vi "Lifter_main.vi"() -> ()   [LabVIEW 2019]
uses:
  LifterSUBVis/Motor Class/Lifter_motor.lvclass
panel:
  out "Step Count":i32
  out "EOS BOS Data":bool
  out "Current insert in the fridge":string
  out "Insert used to calibration":string
  out "Calibration date":string
  out "Motor Speed (rev/s)":dbl
  out "LifterVelocity (mm/s)":dbl
  out "Status bar":string
  out "Moving status":bool
  out "Motor Running":bool
  out "Main Loop Running":bool
  in  "Move to cup abs":bool caption="Move"
  in  "Possition selector":T1(radio)
  in  "stop":bool
  out "chart_temp":waveform(dbl)[](graph)=[{"t0"=timestamp(3772890114.31303 s since 1904-01-01), "dt"=1.0, "Y"=[0.8687935985565186]}, {"t0"=timestamp(3772890114.31303 s since 1904-01-01), "dt"=1.0, "Y"=[86.87935985565186]}, {"t0"=timestamp(3772890114.31303 s since 1904-01-01), "dt"=1.0, "Y"=[30.48853325313992]}, {"t0"=timestamp(3772890114.31303 s since 1904-01-01), "dt"=1.0, "Y"=[303.6385332531399]}]
  out "Step Distance(mm)":dbl
  out "Pot Distance (mm)":dbl format="%#_5g"
  out "L. Limit":bool
  out "U.Limmit":bool
  out "Top":bool
  out "Middle":bool
  out "Bottom":bool
  out "Anneal":bool
  out "Home":bool
  out "Pot":dbl(slide) scale=280.0..-2.0
  out "Possition":dbl(slide) scale=280.0..-2.0
  in  "Show Advance Settings":bool
  in  "Advance Control":enum32{"Page 1", "Beam allignment setup "}(tab)
  in  "Manual Motor direction":bool
  in  "Move to save zone":bool
  in  "Reset Zero":bool
  in  "Up":bool
  in  "Down":bool
  in  "Fine Adjustments (0.005 mm)":dbl min=0.0 max=10.0 step=0.005 format="%#_4g"
  in  "Backlash correction":bool=TRUE
  out "Pot- Step":dbl
  out "ADC Voltage":dbl format="%.5f"
  in  "Move":bool
  in  "Set Velocity":bool
  in  "Set Velocity (mm/s)":dbl min=0.0 max=15.0
  in  "Record data":bool=TRUE
  in  "Remote port":u16=7776
  in  "IP Address":string="192.168.24.142"
  out "Switch Value":dbl
  in  "Data recording interval(ms)":u32=2000
  out "Data wright time (ms)":u32
  in  "Load insert parameters":bool
  in  "initialize the beam allignmet process":bool
  in  "Update newloca tion":bool
  in  "Update the lifter profile":bool
  in  "Insert name":enum16{"Insert #1", "Insert #2", "CALIB_INSERT"}(ring)
  in  "Select the cup":T2(radio)=enum."Bottom Cup on Beam"
  out "Beam alignment is running":bool
  out "New lifter configs_1":dbl[](array[numeric]) caption="Updated lifter configs"
  out "Insert Name_1":string
  out "New lifter configs_2":dbl[](array[numeric]) caption="Updated lifter configs"
  out "Insert Name_2":string
  out "Current insert-lifter config":dbl[](array[numeric]) caption="Updated lifter configs"
  out "Current insert":string
  out "error out":errorcluster
  in  "Exit VI":bool
  # "E-1039 Target Lifter System"
  # "Status"
  # "Possition Controlls"
  # "Cup Possition"
  # "Pot"
  # "Step"
  # "Communication Settings"
  # "Ignore POT and move"
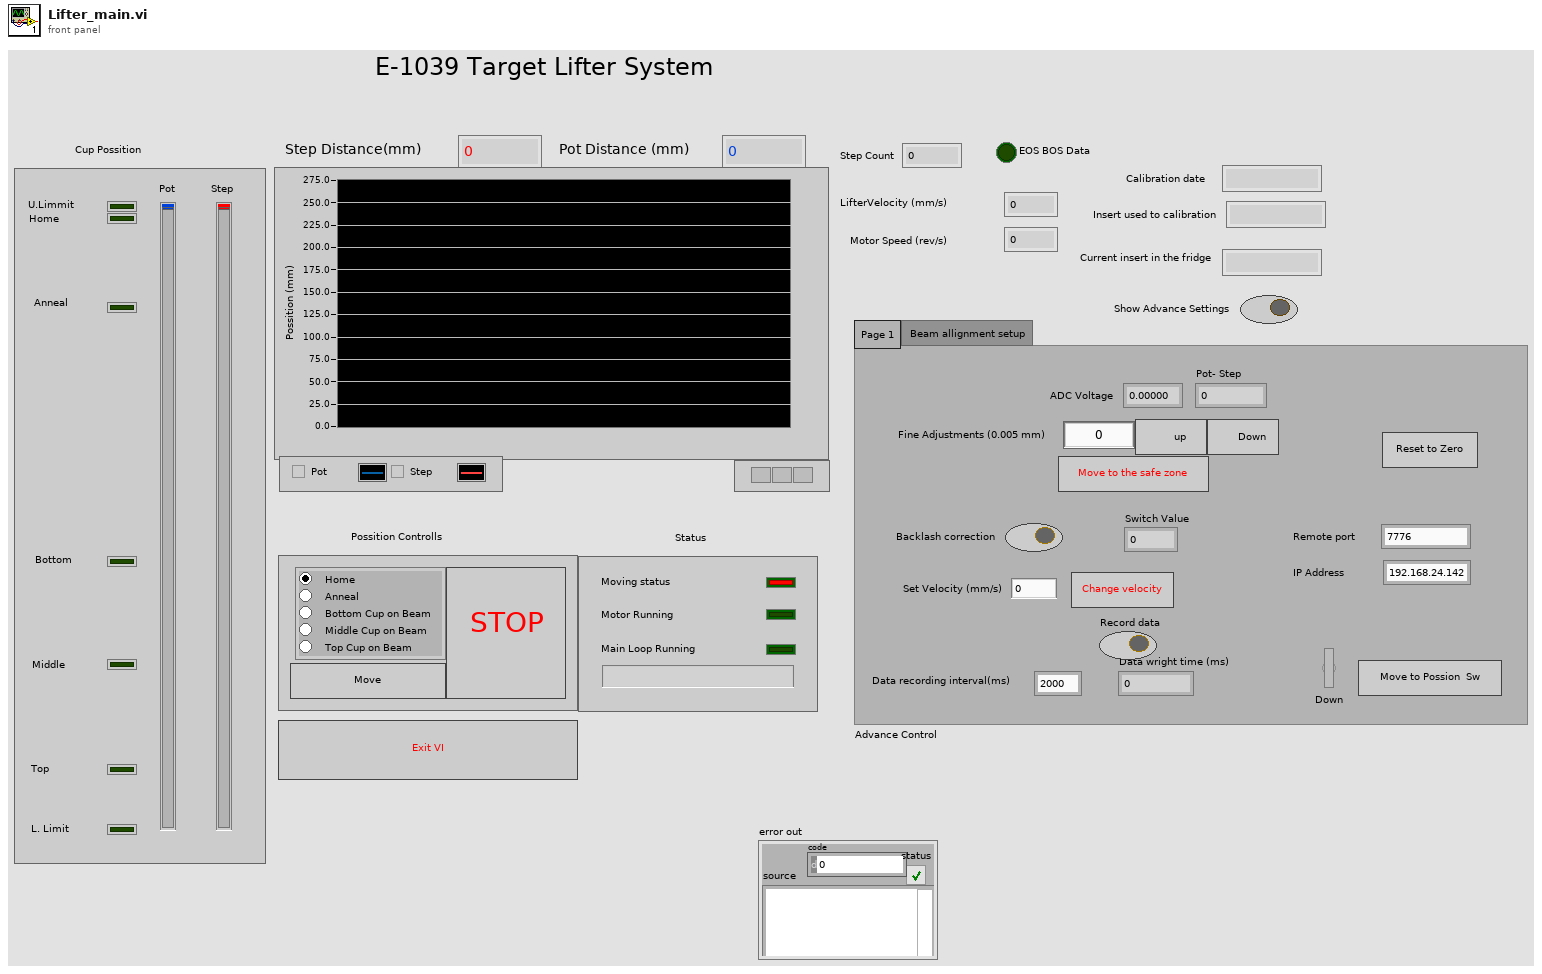
[diagram p1: front panel]
types:
  T1 = enum32{"Home", "Anneal", "Bottom Cup on Beam", "Middle Cup on Beam", "Top Cup on Beam"}
  T2 = enum32{"No Selection", "Bottom Cup on Beam", "Middle Cup on Beam", "Top Cup on Beam"}
  T3 = enum8{"Enabled", "Disabled", "Disabled and Grayed Out"}
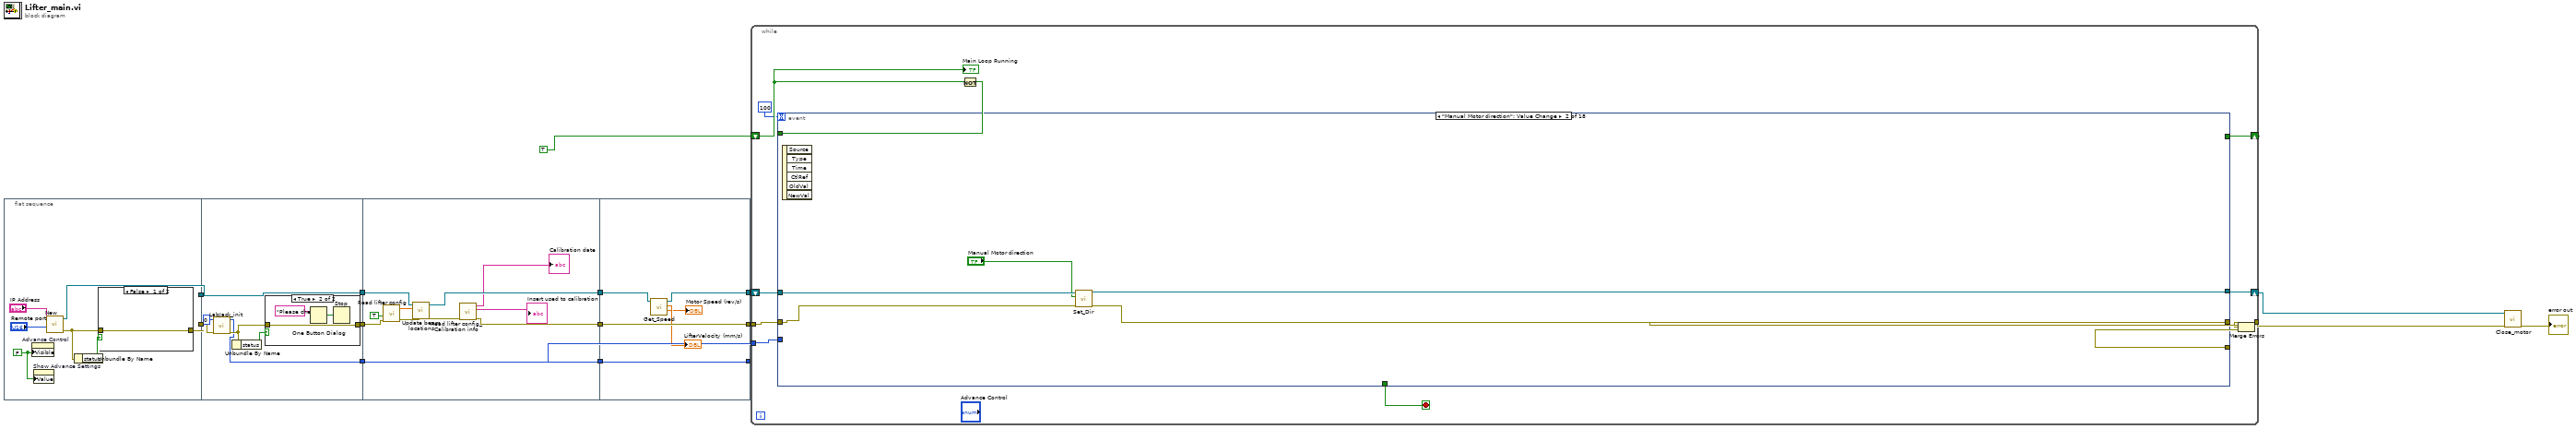
[diagram p0: block diagram]
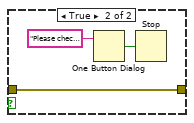
[diagram p2: hidden frame]
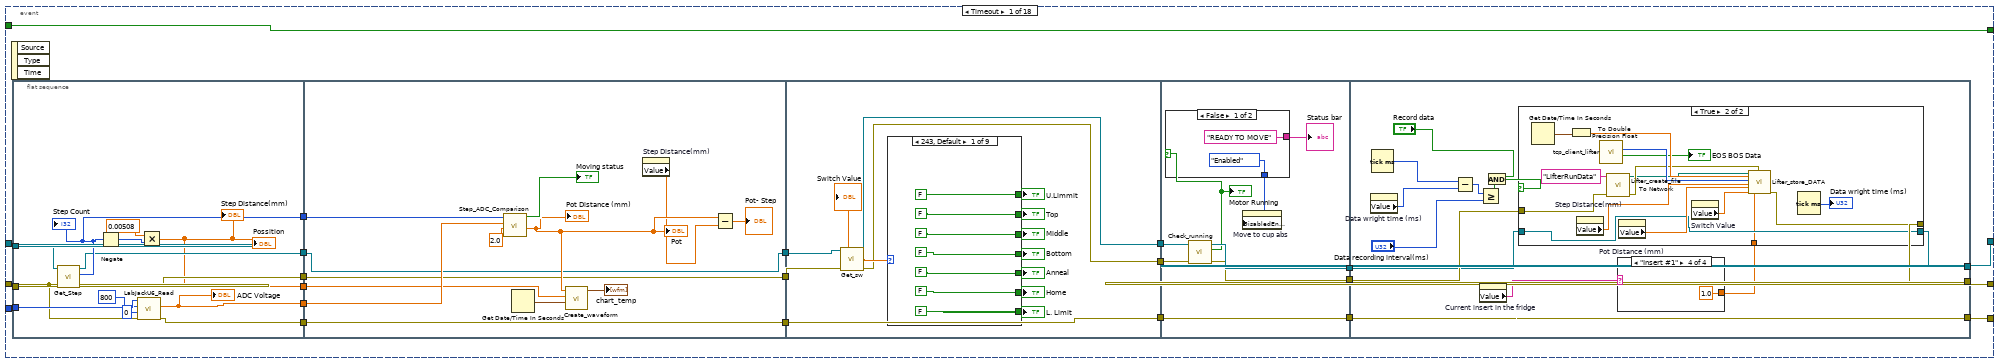
[diagram p4: hidden frame]
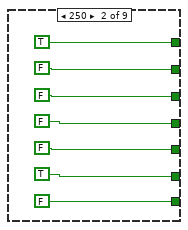
[diagram p5: hidden frame]
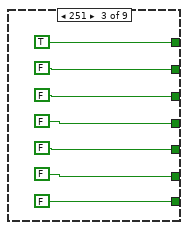
[diagram p6: hidden frame]
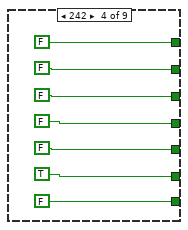
[diagram p7: hidden frame]
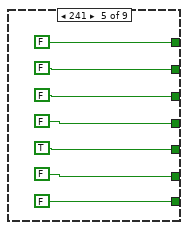
[diagram p8: hidden frame]
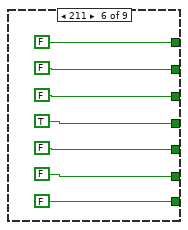
[diagram p9: hidden frame]
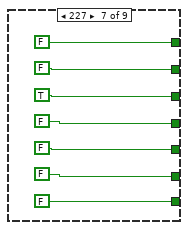
[diagram p10: hidden frame]
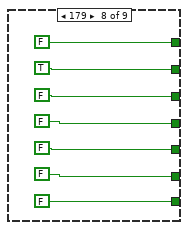
[diagram p11: hidden frame]
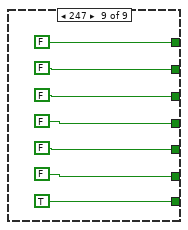
[diagram p12: hidden frame]
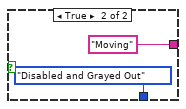
[diagram p13: hidden frame]
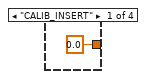
[diagram p14: hidden frame]
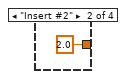
[diagram p15: hidden frame]
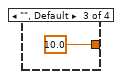
[diagram p16: hidden frame]
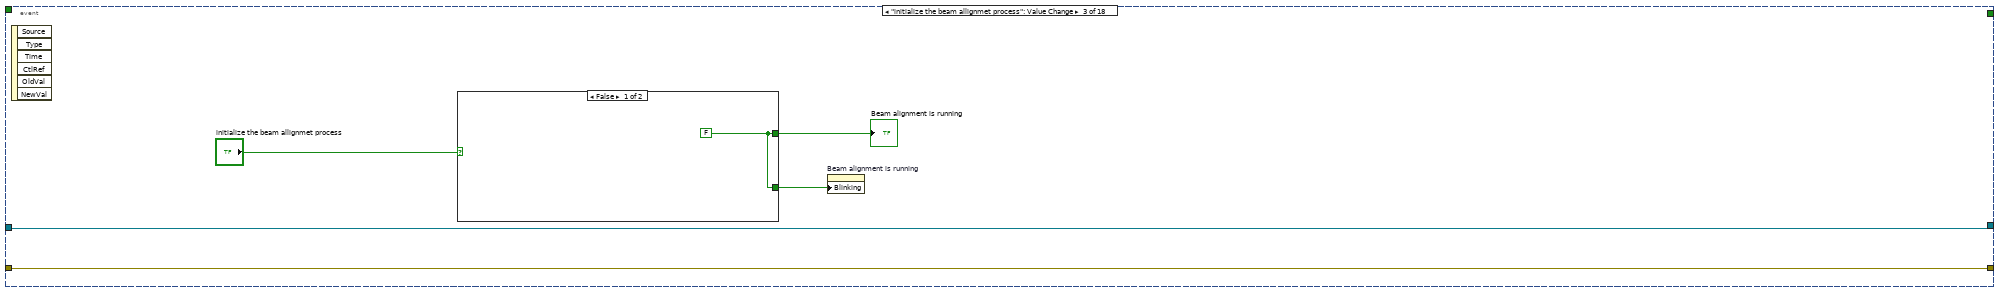
[diagram p18: hidden frame]
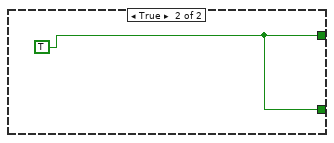
[diagram p19: hidden frame]
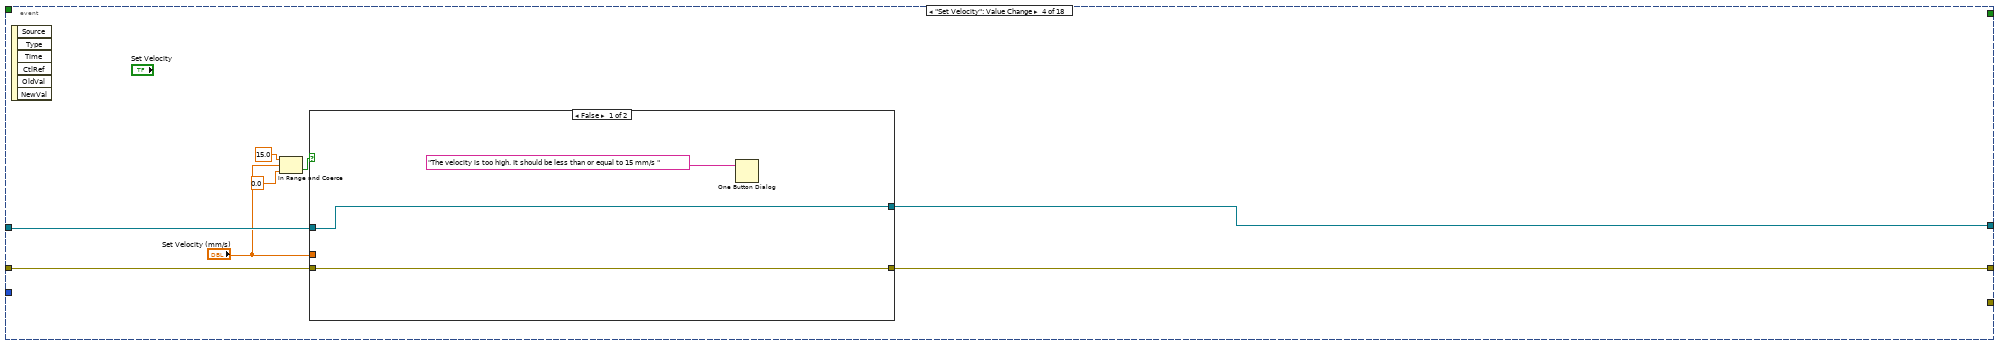
[diagram p20: hidden frame]
diagram:
  n1 = flat-sequence {
    tunnel: [w21] -> w13
    tunnel: [w17] -> w10
    tunnel: w13 -> [w30]
    tunnel: w10 -> [w27]
    tunnel: [w31] -> w6
    tunnel: [w28] -> w4
    tunnel: [w27] -> w2
    tunnel: w6 -> [w47]
    tunnel: [w40] -> w5
    tunnel: w4 -> [w48]
    tunnel: [w48] -> w3
    tunnel: w2 -> [w45]
    tunnel: [w44] -> w1
    tunnel: [w51] -> w11
    tunnel: [w53] -> w12
    tunnel: [w54] -> w14
    tunnel: w5 -> [w54]
    tunnel: w3 -> [w53]
    tunnel: w1 -> [w52]
    frame #0 {
      w16 = FALSE ("Visible")
      n2 = property on="Advance Control" class="TabCtl (strict)"("Visible"=w16) -> ()  [unwired: 2 in, 2 out]
      n3 = property on="Show Advance Settings" class="Bool (strict)"("Value"=w16) -> ()  [unwired: 2 in, 2 out]
      n4 = call "New.vi"("remote port or service name"="Remote port", "address"="IP Address") -> ("error out"=w18:errorcluster, "Lifter_motor out"=w17:refnum<class "Lifter_motor.lvclass">)  [unwired: 8 in]
      n5 = Unbundle By Name(w18) -> ("status"=w22:bool)
      n6 = case shown="False" w22 {
        tunnel: [w23 w25] -> w21
        tunnel: w18 -> [w23 w25]
        frame False {
        }
        frame True {
          n7 = One Button Dialog(message="Please check the motor driver. VI is closing ") -> (true=w24:bool)  [unwired: 1 in]
          n8 = Stop(stop? (T)=w24) -> ()
        }
      }
    }
    frame #1 {
      n9 = call "LabJack_init.vi"("error in"=w30, "Positive Channel #"=0) -> ("error out"=w33:errorcluster, "Handle Out"=w28:i32)  [unwired: 7 in, 1 out]
      n10 = Unbundle By Name(w33) -> ("status"=w32:bool)
      n11 = case shown="True" w32 {
        tunnel: [w34 w36] -> w31
        tunnel: w33 -> [w34 w36]
        frame False {
        }
        frame True {
          n12 = One Button Dialog(message="Please check the ADC. VI is closing ") -> (true=w35:bool)  [unwired: 1 in]
          n13 = Stop(stop? (T)=w35) -> ()
        }
      }
    }
    frame #2 {
      n14 = call "Read lifter config.vi"("Default"=TRUE, "error in (no error)"=w47) -> ("Lifter locations array"=w43:dbl[], "error out"=w46:errorcluster)  [unwired: 5 in]
      n15 = call "Update beam locations.vi"("error in (no error)"=w46, "New cup location"=w43, "Lifter_motor in"=w45) -> ("error out"=w41:errorcluster, "Lifter_motor out"=w44:refnum<class "Lifter_motor.lvclass">)  [unwired: 7 in]
      n16 = call "Read lifter config_Calibration info.vi"("error in (no error)"=w41) -> ("error out"=w40:errorcluster, "Insert"=→"Insert used to calibration":string, "Date"=→"Calibration date":string)  [unwired: 4 in]
    }
    frame #3 {
      n17 = call "Get_Speed.vi"("Lifter_motor in"=w52) -> ("Motor Speed (rev/s)"=→"Motor Speed (rev/s)":dbl, "Target Velocity (mm/s)"=→"LifterVelocity (mm/s)":dbl, "Lifter_motor out"=w51:refnum<class "Lifter_motor.lvclass">)  [unwired: 7 in, 1 out]
    }
  }
  n18 = while {
    tunnel: w14 -> [w65]
    shift-right: [w64] -> _
    shift-left: TRUE ("Main Loop Running") -> [w63]
    tunnel: w12 -> [w60]
    tunnel: [w56] -> w9
    shift-right: [w55] -> w7
    shift-left: w11 -> [w59]
    stop <- w66 stop-if-true
    n19 = Not(x=w63) -> (.not. x?=w62:bool)
    n20 = event shown="[1] \"Manual Motor direction\": Value Change" {
      selector: _ -> [_ _ _ _ _ _ _ _ _ _ _ _ _ _ _ _ _ _]
      dyn-events: _ -> [_ _ _ _ _ _ _ _ _ _ _ _ _ _ _ _ _ _]
      timeout: 100 -> [_ _ _ _ _ _ _ _ _ _ _ _ _ _ _ _ _ _]
      tunnel: [_ _ _ _ _ _ _ _ _ _ _ _ _ _ _ _ w391 _] -> w66
      tunnel: w65 -> [w88 w241 w244 w256 w277 w278 w288 w290 w300 w322 w362 w363 w371 w378 w383 w389 w390 w406]
      tunnel: w62 -> [w87 _ _ _ _ _ _ _ _ _ _ _ _ _ _ _ _ _]
      tunnel: [w87 _ _ _ _ _ _ _ _ _ _ _ _ _ _ _ _ _] -> w64
      tunnel: w60 -> [w78 _ _ _ _ _ _ _ _ _ _ _ _ _ _ _ _ _]
      tunnel: [w81 w239 w244 w254 w271 w278 w282 w289 w299 w322 w361 w364 w370 w377 w382 w388 w390 w407] -> w57
      tunnel: w59 -> [w82 w242 w245 w257 w272 w279 w284 w293 w302 w323 w359 w367 w372 w375 w380 w387 w393 w405]
      tunnel: [w69 w240 w245 w255 w270 w279 w283 w292 w298 w323 w360 w365 w369 w376 w381 w386 w393 w404] -> w55
      tunnel: [w74 _ _ _ _ _ _ _ _ _ w348 _ _ _ _ _ _ _] -> w58
      event Timeout {
        n21 = event-data() -> ()  [unwired: 1 in, 3 out]
        n22 = flat-sequence {
          tunnel: w88 -> [w96]
          tunnel: [w101] -> w86
          tunnel: [w100] -> w83
          tunnel: w82 -> [w99]
          tunnel: [w97] -> w80
          tunnel: [w91] -> w79
          tunnel: w78 -> [w98]
          tunnel: [w95] -> w75
          tunnel: [w90] -> w70
          tunnel: w86 -> [w107]
          tunnel: w83 -> [w102]
          tunnel: w80 -> [w103]
          tunnel: w79 -> [w112]
          tunnel: [w111] -> w76
          tunnel: w75 -> [w111]
          tunnel: w70 -> [w108]
          tunnel: [w103] -> w68
          tunnel: [w102] -> w67
          tunnel: [w118] -> w85
          tunnel: [w117] -> w84
          tunnel: [w115] -> w77
          tunnel: w76 -> [w115]
          tunnel: w68 -> [w120]
          tunnel: w67 -> [w116]
          tunnel: w85 -> [w198]
          tunnel: w84 -> [w197]
          tunnel: w77 -> [w194]
          tunnel: [w196] -> w73
          tunnel: [w195] -> w72
          tunnel: [w194] -> w71
          tunnel: [w216] -> w74
          tunnel: [w215] -> w81
          tunnel: [w205] -> w69
          tunnel: w73 -> [w206]
          tunnel: w72 -> [w214]
          tunnel: w71 -> [w216]
          frame #0 {
            n23 = call "Get_Step.vi"("error in (no error)"=w96, "Lifter_motor in"=w99) -> ("error out"=w97:errorcluster, "Step Count"=w101:i32, "Lifter_motor out"=w100:refnum<class "Lifter_motor.lvclass">)  [unwired: 7 in]
            "Step Count" <- w101
            n24 = Negate(x=w101) -> (-x=w93:i32)
            n25 = call "LabJackU6_Read.vi"("error in"=w96, "Positive Channel #"=0, "n_samples"=800, "Handle In"=w98) -> ("error out"=w95:errorcluster, "Mean ADC Voltage"=w91:dbl)  [unwired: 4 in, 2 out]
            "ADC Voltage" <- w91
            n26 = Multiply(x=0.00508, y=w93) -> (x*y=w90:dbl)
            "Possition" <- w90
            "Step Distance(mm)" <- w90
          }
          frame #1 {
            n27 = call "Step_ADC_Comparison.vi"("Range(mm)"=2.0, "ADC Voltage"=w112, "Steps"=w107) -> ("ADC Distance (mm)"=w106:dbl, "In range"=→"Moving status":bool)  [unwired: 5 in, 1 out]
            "Pot Distance (mm)" <- w106
            "Pot" <- w106
            n28 = Get Date/Time In Seconds() -> (seconds since 1Jan1904=w109:timestamp)
            n29 = call "Create_waveform.vi"("time"=w109, "Step Pos"=w108, "ADC Pos"=w106) -> ("waveform_array"=→"chart_temp":waveform(dbl)[])  [unwired: 8 in]
            n30 = property on="Step Distance(mm)" class="DigNum (strict)"() -> ("Value"=w105:dbl)  [unwired: 2 in, 2 out]
            n31 = Subtract(x=w106, y=w105) -> (x-y=→"Pot- Step":dbl)
          }
          frame #2 {
            n32 = call-dynamic "Get_sw.vi"("error in (no error)"=w120, "Lifter_motor in"=w116) -> ("error out"=w118:errorcluster, "Switch Hex"=w119:dbl, "Lifter_motor out"=w117:refnum<class "Lifter_motor.lvclass">)  [unwired: 7 in]
            "Switch Value" <- w119
            n33 = case shown="243, Default" w119 {
              tunnel: [FALSE ("Lower Limit") TRUE ("Lower Limit") TRUE ("Lower Limit") FALSE ("Lower Limit") FALSE ("Lower Limit") FALSE ("Lower Limit") FALSE ("Lower Limit") FALSE ("Lower Limit") FALSE ("Lower Limit")] -> w127
              tunnel: [FALSE ("Lower Limit") FALSE ("Lower Limit") FALSE ("Lower Limit") FALSE ("Lower Limit") FALSE ("Lower Limit") FALSE ("Lower Limit") FALSE ("Lower Limit") TRUE ("Lower Limit") FALSE ("Lower Limit")] -> w126
              tunnel: [FALSE ("Lower Limit") FALSE ("Lower Limit") FALSE ("Lower Limit") FALSE ("Lower Limit") FALSE ("Lower Limit") FALSE ("Lower Limit") TRUE ("Lower Limit") FALSE ("Lower Limit") FALSE ("Lower Limit")] -> w125
              tunnel: [FALSE ("Lower Limit") FALSE ("Lower Limit") FALSE ("Lower Limit") FALSE ("Lower Limit") FALSE ("Lower Limit") TRUE ("Lower Limit") FALSE ("Lower Limit") FALSE ("Lower Limit") FALSE ("Lower Limit")] -> w124
              tunnel: [FALSE ("Lower Limit") FALSE ("Lower Limit") FALSE ("Lower Limit") FALSE ("Lower Limit") TRUE ("Lower Limit") FALSE ("Lower Limit") FALSE ("Lower Limit") FALSE ("Lower Limit") FALSE ("Lower Limit")] -> w123
              tunnel: [FALSE ("Lower Limit") TRUE ("Lower Limit") FALSE ("Lower Limit") TRUE ("Lower Limit") FALSE ("Lower Limit") FALSE ("Lower Limit") FALSE ("Lower Limit") FALSE ("Lower Limit") FALSE ("Lower Limit")] -> w122
              tunnel: [FALSE ("Lower Limit") FALSE ("Lower Limit") FALSE ("Lower Limit") FALSE ("Lower Limit") FALSE ("Lower Limit") FALSE ("Lower Limit") FALSE ("Lower Limit") FALSE ("Lower Limit") TRUE ("Lower Limit")] -> w121
              frame 243, Default {
              }
              frame 250 {
              }
              frame 251 {
              }
              frame 242 {
              }
              frame 241 {
              }
              frame 211 {
              }
              frame 227 {
              }
              frame 179 {
              }
              frame 247 {
              }
            }
            "L. Limit" <- w121
            "Home" <- w122
            "Bottom" <- w124
            "Middle" <- w125
            "Anneal" <- w123
            "Top" <- w126
            "U.Limmit" <- w127
          }
          frame #3 {
            n34 = call "Check_running.vi"("error in (no error)"=w198, "Lifter_motor in"=w197) -> ("error out"=w195:errorcluster, "Status"=w193:bool, "Lifter_motor out"=w196:refnum<class "Lifter_motor.lvclass">)  [unwired: 6 in, 1 out]
            "Motor Running" <- w193
            n35 = case shown="False" w193 {
              tunnel: [T3."Enabled" ("Disabled") T3."Disabled and Grayed Out" ("Disabled")] -> w192
              tunnel: ["READY TO MOVE" ("Status bar") "Moving" ("Status bar")] -> w191
              frame False {
              }
              frame True {
              }
            }
            "Status bar" <- w191
            n36 = property on="Move to cup abs" class="Bool (strict)"("DisabledEnum"=w192) -> ()  [unwired: 2 in, 2 out]
          }
          frame #4 {
            n37 = property on="Data wright time (ms)" class="DigNum (strict)"() -> ("Value"=w211:u32)  [unwired: 2 in, 2 out]
            n38 = Tick Count (ms)() -> (millisecond timer value=w213:u32)
            n39 = Subtract(x=w213, y=w211) -> (x-y=w212:u32)
            n40 = Greater Or Equal?(x=w212, y="Data recording interval(ms)") -> (x >= y?=w210:bool)
            n41 = property on="Current insert in the fridge" class="Str"() -> ("Value"=w204:string)  [unwired: 2 in, 2 out]
            n42 = And(x="Record data", y=w210) -> (x .and. y?=w209:bool)
            n43 = case shown="\"Insert #1\"" w204 {
              tunnel: [0.0 ("Insert Number") 2.0 ("Insert Number") 10.0 ("Insert Number") 1.0 ("Insert Number")] -> w203
              frame "CALIB_INSERT" {
              }
              frame "Insert #2" {
              }
              frame "", Default {
              }
              frame "Insert #1" {
              }
            }
            n44 = case shown="True" w209 {
              tunnel: w214 -> [w222 w225]
              tunnel: [w222 w233] -> w215
              tunnel: w206 -> [w221 w228]
              tunnel: [w221 w228] -> w205
              tunnel: w203 -> [_ w223]
              frame False {
              }
              frame True {
                n45 = Get Date/Time In Seconds() -> (seconds since 1Jan1904=w237:timestamp)
                n46 = To Double Precision Float(number=w237) -> (double precision float=w236:dbl)
                n47 = property on="Step Distance(mm)" class="DigNum (strict)"() -> ("Value"=w230:dbl)  [unwired: 2 in, 2 out]
                n48 = call "tcp_client_lifter.vi"() -> ("status"=→"EOS BOS Data":bool, "Spill ID"=w235:i32)  [unwired: 8 in, 2 out]
                n49 = call "Lifter_create_file To Network.vi"("error in (no error)"=w225, "File Name"="LifterRunData") -> ("error out"=w227:errorcluster, "dup path"=w226:path)  [unwired: 8 in]
                n50 = property on="Pot Distance (mm)" class="DigNum (strict)"() -> ("Value"=w229:dbl)  [unwired: 2 in, 2 out]
                n51 = property on="Switch Value" class="DigNum (strict)"() -> ("Value"=w234:dbl)  [unwired: 2 in, 2 out]
                n52 = call "Lifter_store_DATA.vi"("file path (dialog if empty)"=w226, "Time stamp"=w236, "Spill ID"=w235, "Step Distance"=w230, "Pot Disance"=w229, "Possition indicator switch"=w234, "Insert Number"=w223, "error in (no error)"=w227) -> ("error out"=w233:errorcluster)  [unwired: 10 in, 1 out]
                n53 = Tick Count (ms)() -> (millisecond timer value=→"Data wright time (ms)":u32)
              }
            }
          }
        }
      }
      event "Manual Motor direction": Value Change {
        n54 = event-data() -> ()  [unwired: 1 in, 6 out]
        n55 = call "Set_Dir.vi"("error in (no error)"=w241, "Direction"="Manual Motor direction", "Lifter_motor in"=w242) -> ("error out"=w239:errorcluster, "Lifter_motor out"=w240:refnum<class "Lifter_motor.lvclass">)  [unwired: 6 in, 1 out]
      }
      event "initialize the beam allignmet process": Value Change {
        n56 = event-data() -> ()  [unwired: 1 in, 6 out]
        n57 = case shown="False" "initialize the beam allignmet process" {
          tunnel: [w248 w249] -> w243
          tunnel: [w248 w249] -> w246
          frame False {
            w248 = FALSE ("Beam alignment is running")
          }
          frame True {
            w249 = TRUE ("Beam alignment is running")
          }
        }
        "Beam alignment is running" <- w243
        n58 = property on="Beam alignment is running" class="Bool (strict)"("Blinking"=w246) -> ()  [unwired: 2 in, 2 out]
      }
      event "Set Velocity": Value Change {
        n59 = event-data() -> ()  [unwired: 1 in, 6 out]
        n60 = In Range and Coerce(upper limit=15.0 ("lower limit"), x="Set Velocity (mm/s)", lower limit=0.0 ("upper limit")) -> (In Range?=w252:bool)  [unwired: 1 out]
        n61 = case shown="False" w252 {
          tunnel: w257 -> [w259 w269]
          tunnel: w256 -> [w260 w268]
          tunnel: [w259 w263] -> w255
          tunnel: [w260 w262] -> w254
          tunnel: "Set Velocity (mm/s)" -> [_ w261]
          frame False {
            n62 = One Button Dialog(message="The velocity is too high. It should be less than or equal to 15 mm/s ") -> ()  [unwired: 1 in, 1 out]
          }
          frame True {
            n63 = call "Set_velocity.vi"("error in (no error)"=w268, "Set Velocity (mm/s)"=w261, "Lifter_motor in"=w269) -> ("error out"=w267:errorcluster, "Lifter_motor out"=w266:refnum<class "Lifter_motor.lvclass">)  [unwired: 7 in]
            n64 = call "Get_Speed.vi"("error in (no error)"=w267, "Lifter_motor in"=w266) -> ("error out"=w262:errorcluster, "Motor Speed (rev/s)"=w264:dbl, "Target Velocity (mm/s)"=w265:dbl, "Lifter_motor out"=w263:refnum<class "Lifter_motor.lvclass">)  [unwired: 6 in]
            n65 = property on="Motor Speed (rev/s)" class="DigNum (strict)"("Value"=w264) -> ()  [unwired: 2 in, 2 out]
            n66 = property on="LifterVelocity (mm/s)" class="DigNum (strict)"("Value"=w265) -> ()  [unwired: 2 in, 2 out]
          }
        }
      }
      event "Move to save zone": Value Change {
        n67 = event-data() -> ()  [unwired: 1 in, 6 out]
        n68 = call "Step mm con.vi"("error in (no error)"=w277, "mm in"=91.054) -> ("error out"=w275:errorcluster, "step out"=w274:i32)  [unwired: 7 in, 1 out]
        n69 = Negate(x=w274) -> (-x=w273:i32)
        n70 = call "Move to Abs Step location.vi"("error in (no error)"=w275, "Absolute step location to move"=w273, "Lifter_motor in"=w272) -> ("error out"=w271:errorcluster, "Lifter_motor out"=w270:refnum<class "Lifter_motor.lvclass">)  [unwired: 6 in, 1 out]
      }
      event "Show Advance Settings": Value Change {
        n71 = event-data() -> ()  [unwired: 1 in, 6 out]
        n72 = property on="Advance Control" class="TabCtl (strict)"("Visible"="Show Advance Settings") -> ()  [unwired: 2 in, 2 out]
      }
      event "Move": Value Change {
        n73 = event-data() -> ()  [unwired: 1 in, 6 out]
        n74 = property on="Step Count" class="DigNum (strict)" props=["Value"]() -> ()  [unwired: 2 in, 3 out]
        n75 = property on="Pot Distance (mm)" class="DigNum (strict)"() -> ("Value"=w286:dbl)  [unwired: 2 in, 2 out]
        n76 = property on="Step Distance(mm)" class="DigNum (strict)"() -> ("Value"=w281:dbl)  [unwired: 2 in, 2 out]
        n77 = property on="Moving status" class="Bool (strict)"() -> ("Value"=w285:bool)  [unwired: 2 in, 2 out]
        n78 = call "Move To Pos.vi"("Lifter_motor in"=w284, "Step In range"=w285, "Step Distance"=w281, "ADC distance"=w286, "Possition selector"="Possition selector", "error in (no error)"=w288) -> ("Lifter_motor out"=w283:refnum<class "Lifter_motor.lvclass">, "error out"=w282:errorcluster)  [unwired: 7 in, 1 out]
      }
      event "Select the cup": Value Change {
        n79 = event-data() -> ()  [unwired: 1 in, 6 out]
        n80 = call "View  beam possitions.vi"("error in (no error)"=w290, "Beam on cup"="Select the cup", "Lifter_motor in"=w293) -> ("error out"=w289:errorcluster, "Lifter_motor out"=w292:refnum<class "Lifter_motor.lvclass">)  [unwired: 6 in, 1 out]
      }
      event "Update the lifter profile": Value Change {
        n81 = event-data() -> ()  [unwired: 1 in, 6 out]
        n82 = property on="Update newloca tion" class="Bool"("DisabledEnum"=T3."Enabled" ("Disabled")) -> ()  [unwired: 2 in, 2 out]
        n83 = property on="Step Distance(mm)" class="DigNum (strict)"() -> ("Value"=w308:dbl)  [unwired: 2 in, 2 out]
        n84 = property on="Select the cup" class="RadioBtnsControl (strict)"() -> ("Value"=w309:T2)  [unwired: 2 in, 2 out]
        n85 = call "Generate_insert cup locations .vi"("Lifter reading (mm)"=w308, "Select the cup"=w309) -> ("Top"=w305:dbl, "Middle"=w306:dbl, "Bottom"=w307:dbl)  [unwired: 7 in]
        n86 = call "Write to lifter config.vi"("Insert name"="Insert name", "Bottom"=w307, "Middle"=w306, "Top"=w305, "error in (no error)"=w300) -> ("error out"=w303:errorcluster)  [unwired: 9 in, 1 out]
        n87 = call "Write to lifter config.vi"("Default"=TRUE, "Bottom"=w307, "Middle"=w306, "Top"=w305, "error in (no error)"=w303) -> ("Cup locations"=w294:dbl[], "error out"=w301:errorcluster)  [unwired: 9 in]
        "Current insert-lifter config" <- w294
        n88 = property on="Insert name" class="Enum (strict)"() -> ("Strings []"=w296:string[])  [unwired: 2 in, 2 out]
        n89 = Index Array(array=w296, index="Insert name") -> (element=→"Current insert":string)
        n90 = call "Update beam locations.vi"("error in (no error)"=w301, "New cup location"=w294, "Lifter_motor in"=w302) -> ("error out"=w299:errorcluster, "Lifter_motor out"=w298:refnum<class "Lifter_motor.lvclass">)  [unwired: 7 in]
      }
      event "Update newloca tion": Value Change {
        n91 = event-data() -> ()  [unwired: 1 in, 6 out]
        n92 = property on="Insert name" class="Enum (strict)"() -> ("Value"=w317:enum16{"Insert #1", "Insert #2", "CALIB_INSERT"})  [unwired: 2 in, 2 out]
        n93 = call "Read inserts profiles.vi"("Insert name"=w317) -> ("error out"=w344:errorcluster, "top cup length"=w330:dbl)  [unwired: 7 in]
        n94 = Increment(x=w317) -> (x+1=w315:enum16{"Insert #1", "Insert #2", "CALIB_INSERT"})
        n95 = call "Read inserts profiles.vi"("error in (no error)"=w344, "Insert name"=w315) -> ("error out"=w342:errorcluster, "top cup length"=w343:dbl)  [unwired: 6 in]
        n96 = Subtract(x=w330, y=w343) -> (x-y=w340:dbl)
        n97 = property on="Insert name" class="Enum (strict)"() -> ("Strings []"=w316:string[])  [unwired: 2 in, 2 out]
        n98 = call "Read lifter config.vi"("Insert name"=w317, "error in (no error)"=w342) -> ("Lifter locations array"=w341:dbl[], "error out"=w332:errorcluster)  [unwired: 5 in]
        n99 = Add(x=w340, y=w341) -> (x+y=w339:dbl[])
        "New lifter configs_1" <- w339
        n100 = Index Array(array=w316, index=w315) -> (element=→"Insert Name_1":string)
        n101 = Index Array(array=w339, index #1=0 ("index")) -> (element #1=w338:dbl, element #2=w337:dbl, element #3=w336:dbl)  [unwired: 2 in]
        n102 = call "Write to lifter config.vi"("Insert name"=w315, "Bottom"=w338, "Middle"=w337, "Top"=w336) -> ()  [unwired: 10 in, 2 out]
        n103 = Increment(x=w315) -> (x+1=w312:enum16{"Insert #1", "Insert #2", "CALIB_INSERT"})
        n104 = call "Read inserts profiles.vi"("error in (no error)"=w332, "Insert name"=w312) -> ("error out"=w331:errorcluster, "top cup length"=w335:dbl)  [unwired: 6 in]
        n105 = Subtract(x=w330, y=w335) -> (x-y=w333:dbl)
        n106 = property on="Insert name" class="Enum (strict)"() -> ("Strings []"=w313:string[])  [unwired: 2 in, 2 out]
        n107 = call "Read lifter config.vi"("Insert name"=w317, "error in (no error)"=w331) -> ("Lifter locations array"=w334:dbl[], "error out"=w320:errorcluster)  [unwired: 5 in]
        n108 = Index Array(array=w313, index=w312) -> (element=→"Insert Name_2":string)
        n109 = Add(x=w333, y=w334) -> (x+y=w326:dbl[])
        "New lifter configs_2" <- w326
        n110 = Index Array(array=w326, index #1=0 ("index")) -> (element #1=w327:dbl, element #2=w328:dbl, element #3=w329:dbl)  [unwired: 2 in]
        n111 = call "Write to lifter config.vi"("Insert name"=w312, "Bottom"=w327, "Middle"=w328, "Top"=w329, "error in (no error)"=w320) -> ("error out"=w321:errorcluster)  [unwired: 9 in, 1 out]
        n112 = case shown="\"Insert #1\", Default" w317 {
          tunnel: ["INSERT_1" ("section") "INSERT_2" ("section") "CALIB_INSERT" ("section")] -> w318
          frame "Insert #1", Default {
          }
          frame "Insert #2" {
          }
          frame "CALIB_INSERT" {
          }
        }
        n113 = Get Date/Time String() -> (date string=w319:string)  [unwired: 3 in, 1 out]
        n114 = call "Write to lifter config_Calibration info.vi"("error in (no error)"=w321, "Insert"=w318, "Date"=w319) -> ()  [unwired: 6 in, 1 out]
      }
      event "Load insert parameters": Value Change {
        n115 = event-data() -> ()  [unwired: 1 in, 6 out]
        n116 = property on="Insert name" class="Enum (strict)"() -> ("Value"=w357:enum16{"Insert #1", "Insert #2", "CALIB_INSERT"})  [unwired: 2 in, 2 out]
        n117 = call "Read lifter config.vi"("Insert name"=w357) -> ("Lifter locations array"=w353:dbl[], "error out"=w356:errorcluster)  [unwired: 6 in]
        n118 = property on="Insert name" class="Enum (strict)"() -> ("Strings []"=w358:string[])  [unwired: 2 in, 2 out]
        n119 = Index Array(array=w358, index=w357) -> (element=w355:string)
        "Current insert in the fridge" <- w355
        n120 = call "Update beam locations.vi"("error in (no error)"=w362, "New cup location"=w353, "Lifter_motor in"=w359) -> ("error out"=w361:errorcluster, "Lifter_motor out"=w360:refnum<class "Lifter_motor.lvclass">)  [unwired: 7 in]
        n121 = call "Write to lifter config_Running info.vi"("error in (no error)"=w356, "Insert Name"=w355) -> ("error out"=w349:errorcluster)  [unwired: 7 in]
        n122 = Index Array(array=w353) -> (element #1=w352:dbl, element #2=w351:dbl, element #3=w350:dbl)  [unwired: 3 in]
        n123 = call "Write to lifter config.vi"("Default"=TRUE, "Bottom"=w352, "Middle"=w351, "Top"=w350, "error in (no error)"=w349) -> ("error out"=w348:errorcluster)  [unwired: 9 in, 1 out]
      }
      event "Move to cup abs": Value Change {
        n124 = event-data() -> ()  [unwired: 1 in, 6 out]
        n125 = property on="Possition selector" class="RadioBtnsControl (strict)"() -> ("Value"=w366:T1)  [unwired: 2 in, 2 out]
        n126 = property on="Moving status" class="Bool (strict)"() -> ("Value"=w368:bool)  [unwired: 2 in, 2 out]
        n127 = call "Move To Abs sw.vi"("error in (no error)"=w363, "Step In range"=w368, "Possition selector"=w366, "Lifter_motor in"=w367) -> ("error out"=w364:errorcluster, "Lifter_motor out"=w365:refnum<class "Lifter_motor.lvclass">)  [unwired: 6 in]
      }
      event "Backlash correction": Value Change {
        n128 = event-data() -> ()  [unwired: 1 in, 6 out]
        n129 = call "Turn on_off backlash correction.vi"("error in (no error)"=w371, "Backlash correction"="Backlash correction", "Lifter_motor in"=w372) -> ("error out"=w370:errorcluster, "Lifter_motor out"=w369:refnum<class "Lifter_motor.lvclass">)  [unwired: 7 in]
      }
      event "Up": Value Change {
        n130 = event-data() -> ()  [unwired: 1 in, 6 out]
        n131 = call "Move_mm_abs.vi"("error in (no error)"=w378, "mm"="Fine Adjustments (0.005 mm)", "Lifter_motor in"=w375) -> ("error out"=w377:errorcluster, "Lifter_motor out"=w376:refnum<class "Lifter_motor.lvclass">)  [unwired: 7 in]
      }
      event "Down": Value Change {
        n132 = event-data() -> ()  [unwired: 1 in, 6 out]
        n133 = property on="Fine Adjustments (0.005 mm)" class="DigNum (strict)"() -> ("Value"=w385:dbl)  [unwired: 2 in, 2 out]
        n134 = Multiply(x=w385, y=-1.0) -> (x*y=w379:dbl)
        n135 = call "Move_mm_abs.vi"("error in (no error)"=w383, "mm"=w379, "Lifter_motor in"=w380) -> ("error out"=w382:errorcluster, "Lifter_motor out"=w381:refnum<class "Lifter_motor.lvclass">)  [unwired: 7 in]
      }
      event "stop": Value Change {
        n136 = event-data() -> ()  [unwired: 1 in, 6 out]
        n137 = call "Motor_Stop.vi"("error in (no error)"=w389, "Lifter_motor in"=w387) -> ("error out"=w388:errorcluster, "Lifter_motor out"=w386:refnum<class "Lifter_motor.lvclass">)  [unwired: 7 in, 1 out]
      }
      event "Exit VI": Value Change {
        n138 = event-data() -> ()  [unwired: 1 in, 6 out]
        n139 = property on="Motor Running" class="Bool (strict)"() -> ("Value"=w392:bool)  [unwired: 2 in, 2 out]
        n140 = case shown="False" w392 {
          tunnel: [w394 FALSE] -> w391
          frame False {
            n141 = Two Button Dialog(message="Do you really need to close the VI ") -> (T button?=w395:bool)  [unwired: 2 in]
            n142 = case shown="False" w395 {
              tunnel: [FALSE TRUE] -> w394
              frame False {
              }
              frame True {
              }
            }
          }
          frame True {
            n143 = One Button Dialog(message="Please wait. The lifter is still moving") -> ()  [unwired: 1 in, 1 out]
          }
        }
      }
      event "Reset Zero": Value Change {
        n144 = event-data() -> ()  [unwired: 1 in, 6 out]
        n145 = Two Button Dialog(message="Do You need to Rest the motor controller ? are you sure?", 2:"Yes" ("T button name (\"OK\")")) -> (T button?=w401:bool)  [unwired: 1 in]
        n146 = case shown="True" w401 {
          tunnel: [w408 w414] -> w407
          tunnel: w406 -> [w408 w413]
          tunnel: w405 -> [w409 w411]
          tunnel: [w409 w410] -> w404
          frame False {
          }
          frame True {
            n147 = call "Set_Step.vi"("error in (no error)"=w413, "Set_stepcount"=0, "Lifter_motor in"=w411) -> ("error out"=w414:errorcluster, "Lifter_motor out"=w410:refnum<class "Lifter_motor.lvclass">)  [unwired: 7 in]
          }
        }
      }
    }
    n148 = Merge Errors(w57, w58) -> (w56:errorcluster)
    "Main Loop Running" <- w63
  }
  n149 = call "Close_motor.vi"("error in (no error)"=w9, "Lifter_motor in"=w7) -> ("error out"=→"error out":errorcluster)  [unwired: 9 in]
